vi "String to U64.vi"(11 "String":string) -> (2 "length":i32, 3 "U64":u64 format="%016x")   [LabVIEW 2024]
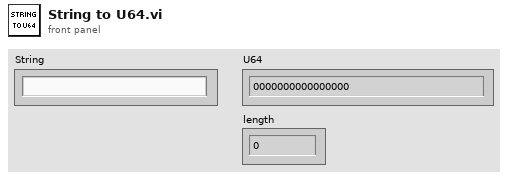
[diagram p1: front panel]
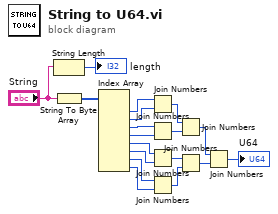
[diagram p0: block diagram]
diagram:
  n1 = String Length(string="String") -> (length=→"length":i32)
  n2 = String To Byte Array(string="String") -> (unsigned byte array=w18:u8[])
  n3 = Index Array(array=w18) -> (element #1=w14:u8, element #2=w15:u8, element #3=w12:u8, element #4=w11:u8, element #5=w7:u8, element #6=w6:u8, element #7=w5:u8, element #8=w4:u8)  [unwired: 8 in]
  n4 = Join Numbers(hi=w14, lo=w15) -> ((hi.lo)=w13:u16)
  n5 = Join Numbers(hi=w12, lo=w11) -> ((hi.lo)=w10:u16)
  n6 = Join Numbers(hi=w7, lo=w6) -> ((hi.lo)=w8:u16)
  n7 = Join Numbers(hi=w5, lo=w4) -> ((hi.lo)=w9:u16)
  n8 = Join Numbers(hi=w13, lo=w10) -> ((hi.lo)=w3:u32)
  n9 = Join Numbers(hi=w8, lo=w9) -> ((hi.lo)=w2:u32)
  n10 = Join Numbers(hi=w3, lo=w2) -> ((hi.lo)=→"U64":u64)
